vi "R1Master.vi"(6 "LabVIEW Web Service":refnum<class "Web Service.lvclass">=refnum) -> ()   [LabVIEW 2016]
uses:
  <vilib>/wsapi/Web Service.lvclass
  Controls/pH_SetParams Standard.ctl
  Controls/R1SBR_SetParams.ctl
  <vilib>/Platform/TimedLoop/XDataNode/timing_clust.ctl
  <vilib>/Platform/TimedLoop/XDataNode/nitl_modes.ctl
  <vilib>/Platform/TimedLoop/XDataNode/wakeup.ctl
  Controls/pH_Manual Standard.ctl
  <vilib>/Platform/TimedLoop/XDataNode/loadnilvce.vi
  <vilib>/Platform/TimedLoop/XDataNode/XDataNode.xnode
  <vilib>/Platform/TimedLoop/XDataNode/XDNodeRunTimeDep.lvlib
panel:
  out "ORP, V":dbl
  in  "R1SBR_SetParams":T1=[{"Phase"="Plug Feed", "Time, min"=60.0, "SBR_Manual"={"Media Pump"=TRUE, "Water Pump"=TRUE, "Effluent Pump"=FALSE, "Release Valve"=FALSE, "Gas Pump"=FALSE}}, {"Phase"="Mixed Feed", "Time, min"=80.0, "SBR_Manual"={"Media Pump"=TRUE, "Water Pump"=TRUE, "Effluent Pump"=FALSE, "Release Valve"=FALSE, "Gas Pump"=TRUE}}, {"Phase"="Mixed W/O Feed", "Time, min"=0.0, "SBR_Manual"={"Media Pump"=FALSE, "Water Pump"=FALSE, "Effluent Pump"=FALSE, "Release Valve"=FALSE, "Gas Pump"=TRUE}}, {"Phase"="Settle", "Time, min"=10.0, "SBR_Manual"={"Media Pump"=FALSE, "Water Pump"=FALSE, "Effluent Pump"=FALSE, "Release Valve"=FALSE, "Gas Pump"=FALSE}}, {"Phase"="Decant", "Time, min"=4.0, "SBR_Manual"={"Media Pump"=FALSE, "Water Pump"=FALSE, "Effluent Pump"=TRUE, "Release Valve"=TRUE, "Gas Pump"=FALSE}}, {"Phase"="Idle", "Time, min"=1.0, "SBR_Manual"={"Media Pump"=FALSE, "Water Pump"=FALSE, "Effluent Pump"=FALSE, "Release Valve"=FALSE, "Gas Pump"=FALSE}}] {"Time, min" min=1.0}
  out "error out Na":errorcluster
  out "error Out NH4 Nh4":errorcluster
  out "error out":errorcluster
  out "replace with nh4 set params":T2={"Set Point, mg/L"=0.0, "Tolerance, mg/L"=0.05, "N2 Valve Gain"=5000.0, "Air Valve Gain"=1000.0}
  in  "R1NH4Manual":cluster{"NH4 Pump Flowrate, ml/min":dbl}
  out "replace with nh4 switch":bool=TRUE
  in  "R1DOSetParams 2":T2={"Set Point, mg/L"=0.0, "Tolerance, mg/L"=0.05, "N2 Valve Gain"=5000.0, "Air Valve Gain"=1000.0}
  in  "R1 NH4_Switch":bool=TRUE
  out "add NH4 NA probes":cluster{"Signal":dbl, "Value":dbl}={"Signal"=0.0006045842747169349, "Value"=-0.0019895042131602755}
  out "error out (DATA COLLECT)":errorcluster
  out "error out (SBR)":errorcluster
  out "Graph":T3(graph)={"Value"=-0.0019895042131602755, "Value, UNITS HERE"=0.0, "Value"=8.00229484709635}
  in  "R1SBRManual":T4
  in  "R1 SBR_Switch":bool
  in  "R1DOSetParams":T2={"Set Point, mg/L"=0.25, "Tolerance, mg/L"=0.025, "N2 Valve Gain"=200.0, "Air Valve Gain"=1050.0}
  in  "R1DOManual":cluster{"Air MFC":dbl, "N2 MFC":dbl} {"Air MFC" scale=0.0..500.0; "N2 MFC" scale=0.0..500.0}
  in  "R1 DO_Switch":bool=TRUE
  out "R1DO":cluster{"Signal":dbl, "Value":dbl}={"Signal"=0.0006045842747169349, "Value"=-0.0019895042131602755}
  in  "R1 pH_Switch":bool=TRUE
  in  "R1pH_SetParams":T5={"Set Point"=8.0, "Tolerance"=0.1, "Pump Time On, secs"=6.0}
  in  "R1pH_Manual":cluster{"Acid Pump":bool, "Base Pump":bool}
  out "pH":cluster{"Signal":dbl, "Value":dbl}={"Signal"=0.013505965504601244, "Value"=8.00229484709635}
  out "Timestamp":string="03/16/2018 18:24:55.540"
  out "Status":string="Off"
  out "Cycle Time Elapsed":dbl
  out "Phase Time Elapsed":dbl
  # "Don't press the run button!"
  # "Use the web service input terminal to call the VIs on the Service subpalette of the Web Services palette. Do not remove it from the connector pane unless you don't need access to the palette."
  # "Any additional terminals added to the connector pane of a startup VI will be ignored."
  # "Don't press the run button!"
  # "SBR Control"
  # "If On, Automate SBR Cycle"
  # "DO Control"
  # "pH Control"
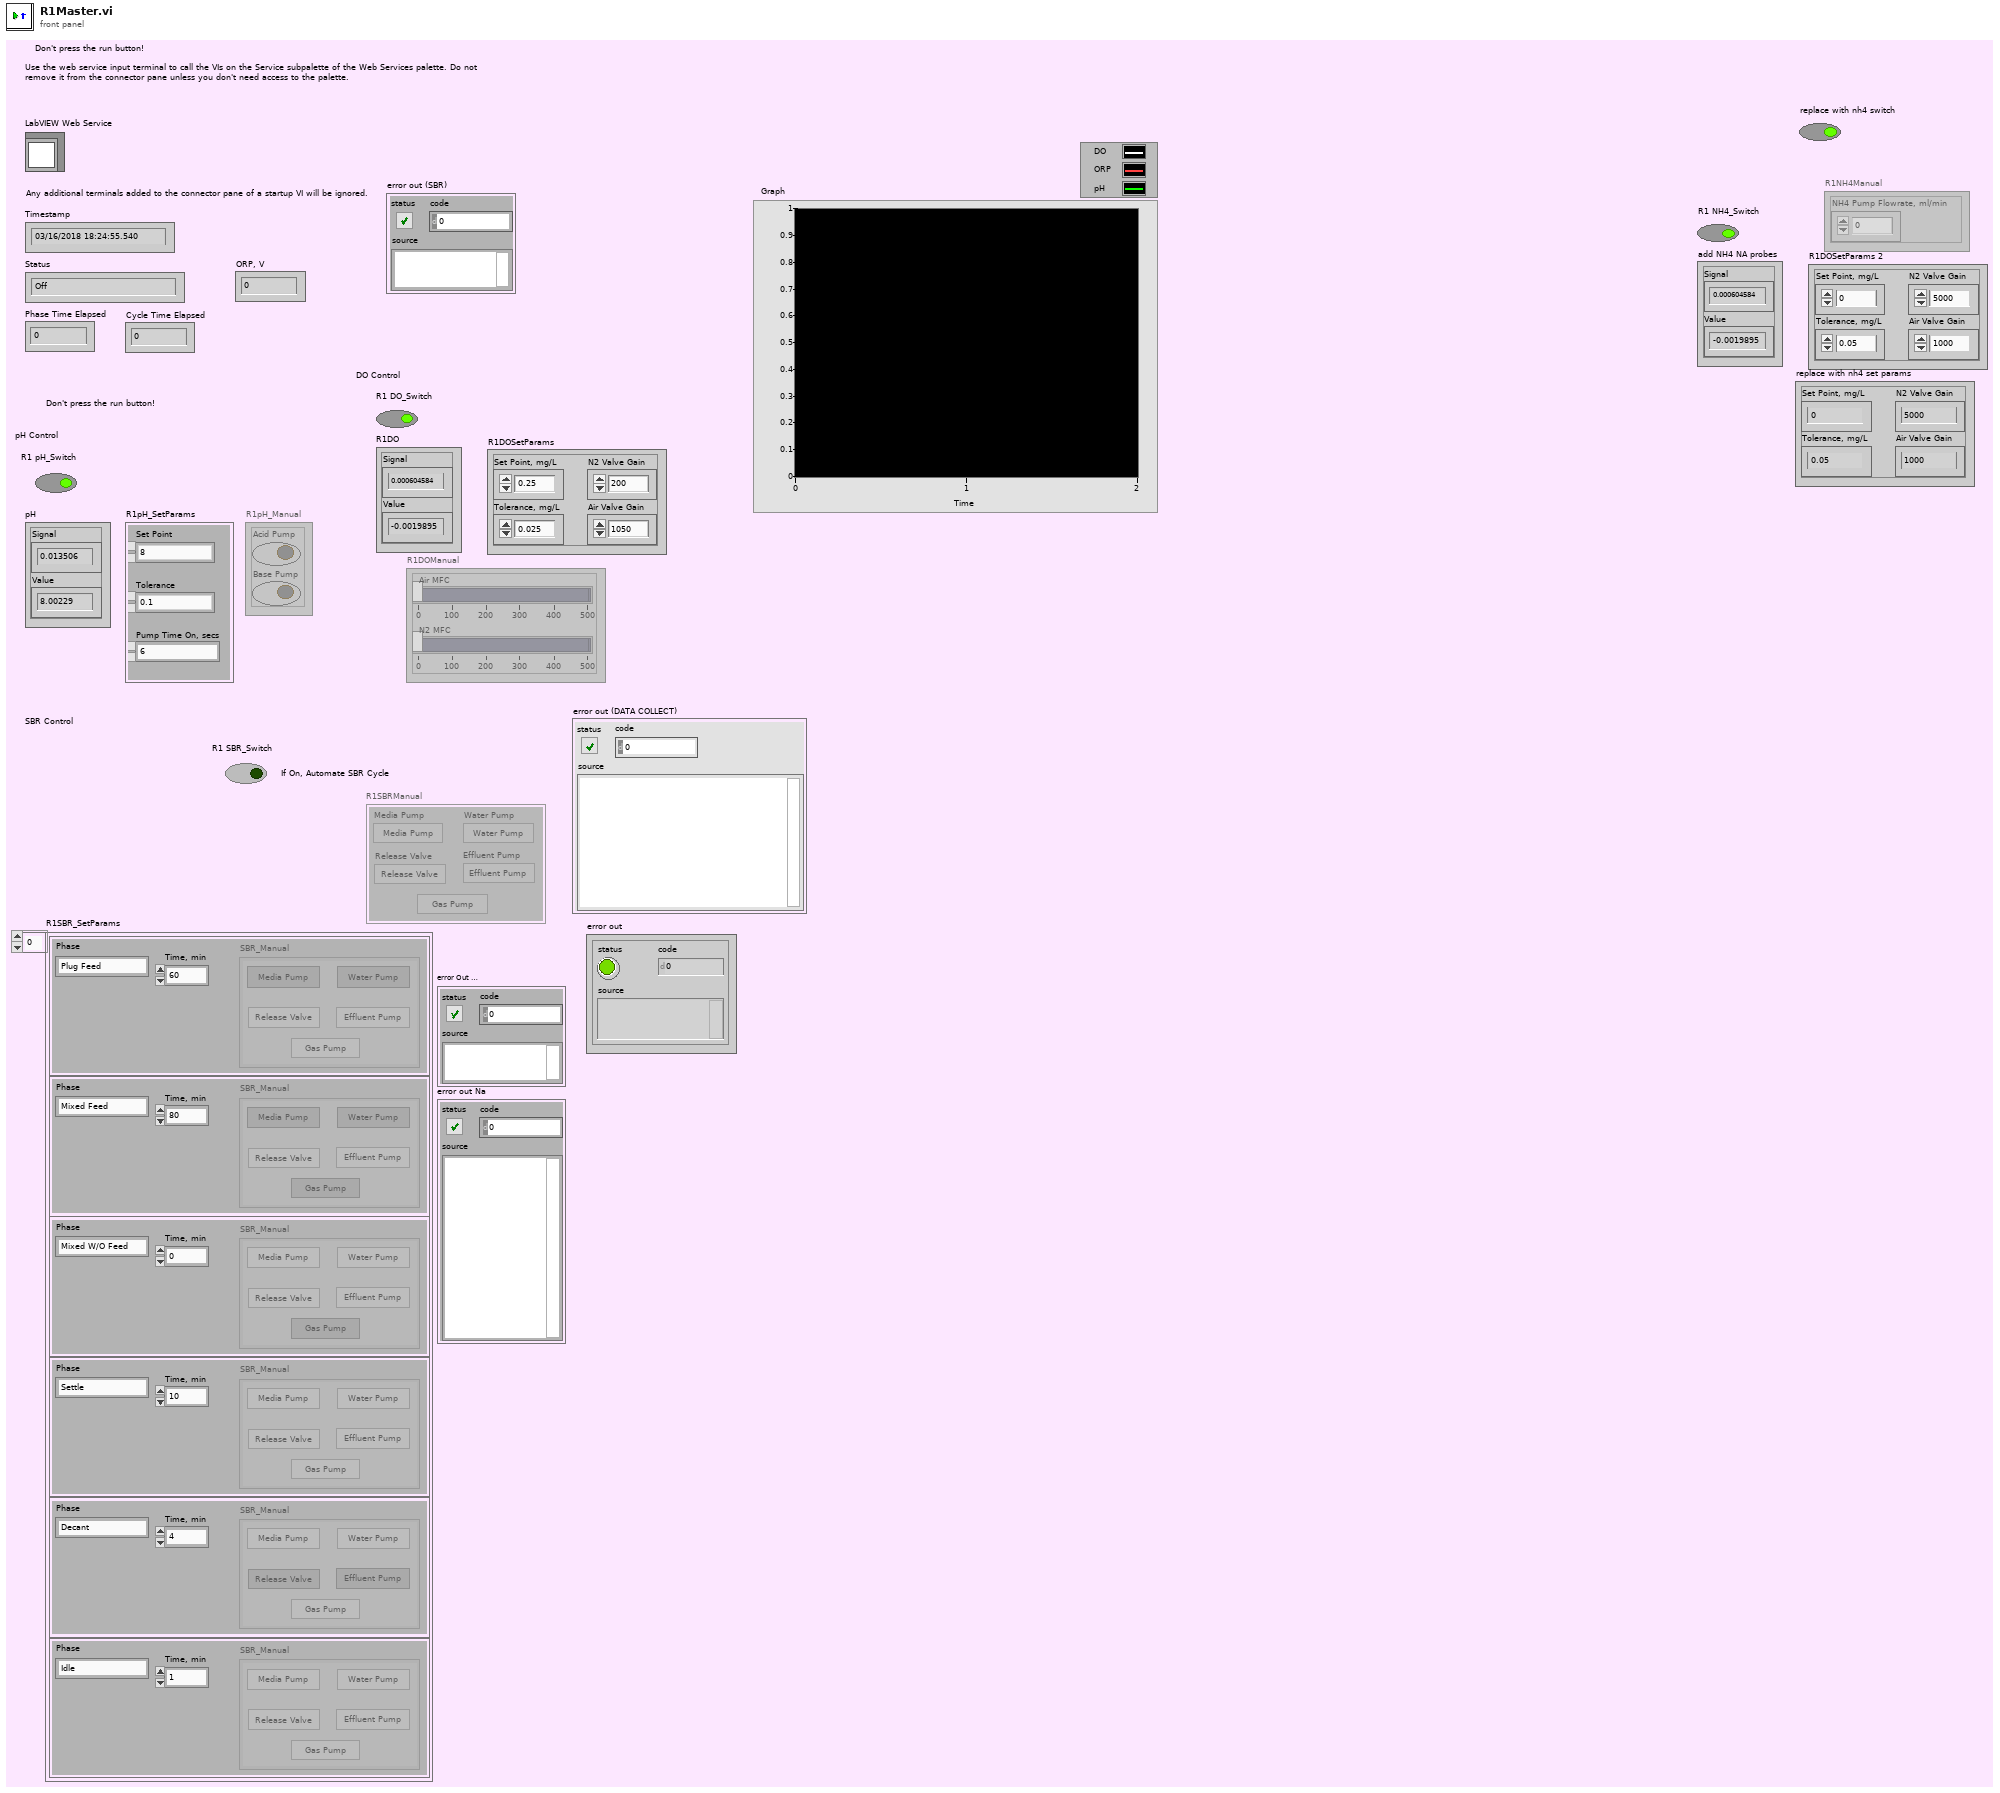
[diagram p1: front panel]
types:
  T1 = typedef "R1SBR_SetParams.ctl" = cluster{"Phase":string, "Time, min":dbl, "SBR_Manual":cluster{"Media Pump":bool, "Water Pump":bool, "Effluent Pump":bool, "Release Valve":bool, "Gas Pump":bool}}[]
  T2 = cluster{"Set Point, mg/L":dbl, "Tolerance, mg/L":dbl, "N2 Valve Gain":dbl, "Air Valve Gain":dbl}
  T3 = cluster{"Value":dbl, "Value, UNITS HERE":dbl, "Value":dbl}
  T4 = cluster{"Media Pump":bool, "Water Pump":bool, "Effluent Pump":bool, "Release Valve":bool, "Gas Pump":bool}
  T5 = typedef "pH_SetParams Standard.ctl" = cluster{"Set Point":dbl, "Tolerance":dbl, "Pump Time On, secs":dbl}
  T6 = typedef "XDNodeRunTimeDep.lvlib/timing_clust.ctl" = cluster{"Expected End [f-1]":u64, "Actual End [f-1]":u64, "Finished Late? [f-1]":bool, "Expected End [i-1]":u64, "Actual End [i-1]":u64, "Finished Late? [i-1]":bool, "Expected Start [i]":u64, "Actual Start [i]":u64, "Expected Start [f]":u64, "Actual Start [f]":u64, "Source Name":string, "Structure Name":string, "Period":i64, "Deadline":i64, "Offset":i64, "Start":i64, "Priority":i32, "Timeout":i32, "Mode":T7, "Wakeup Reason":T8, "Error":errorcluster, "Source Type":string, "Secondary Source Type":string, "Global End Time":u64, "Global Start Time":u64, "Frame Duration":u64, "Iteration Duration":u64, "Assigned CPU":i32, "I/O Scan Engine Mode":u32}
  T7 = typedef "XDNodeRunTimeDep.lvlib/nitl_modes.ctl" = enum32{"No Change", "Process missed periods, maintain original phase", "Discard missed periods, maintain original phase", "Process missed periods, ignore original phase", "Discard missed periods, ignore original phase"}
  T8 = typedef "XDNodeRunTimeDep.lvlib/wakeup.ctl" = enum32{"Normal", "Aborted", "Asynchronous wakeup", "Timing source error", "Timed loop error", "Timeout"}
  T9 = enum8{"Enabled", "Disabled", "Disabled and Grayed Out"}
  T10 = typedef "pH_Manual Standard.ctl" = cluster{"Acid Pump":bool, "Base Pump":bool}
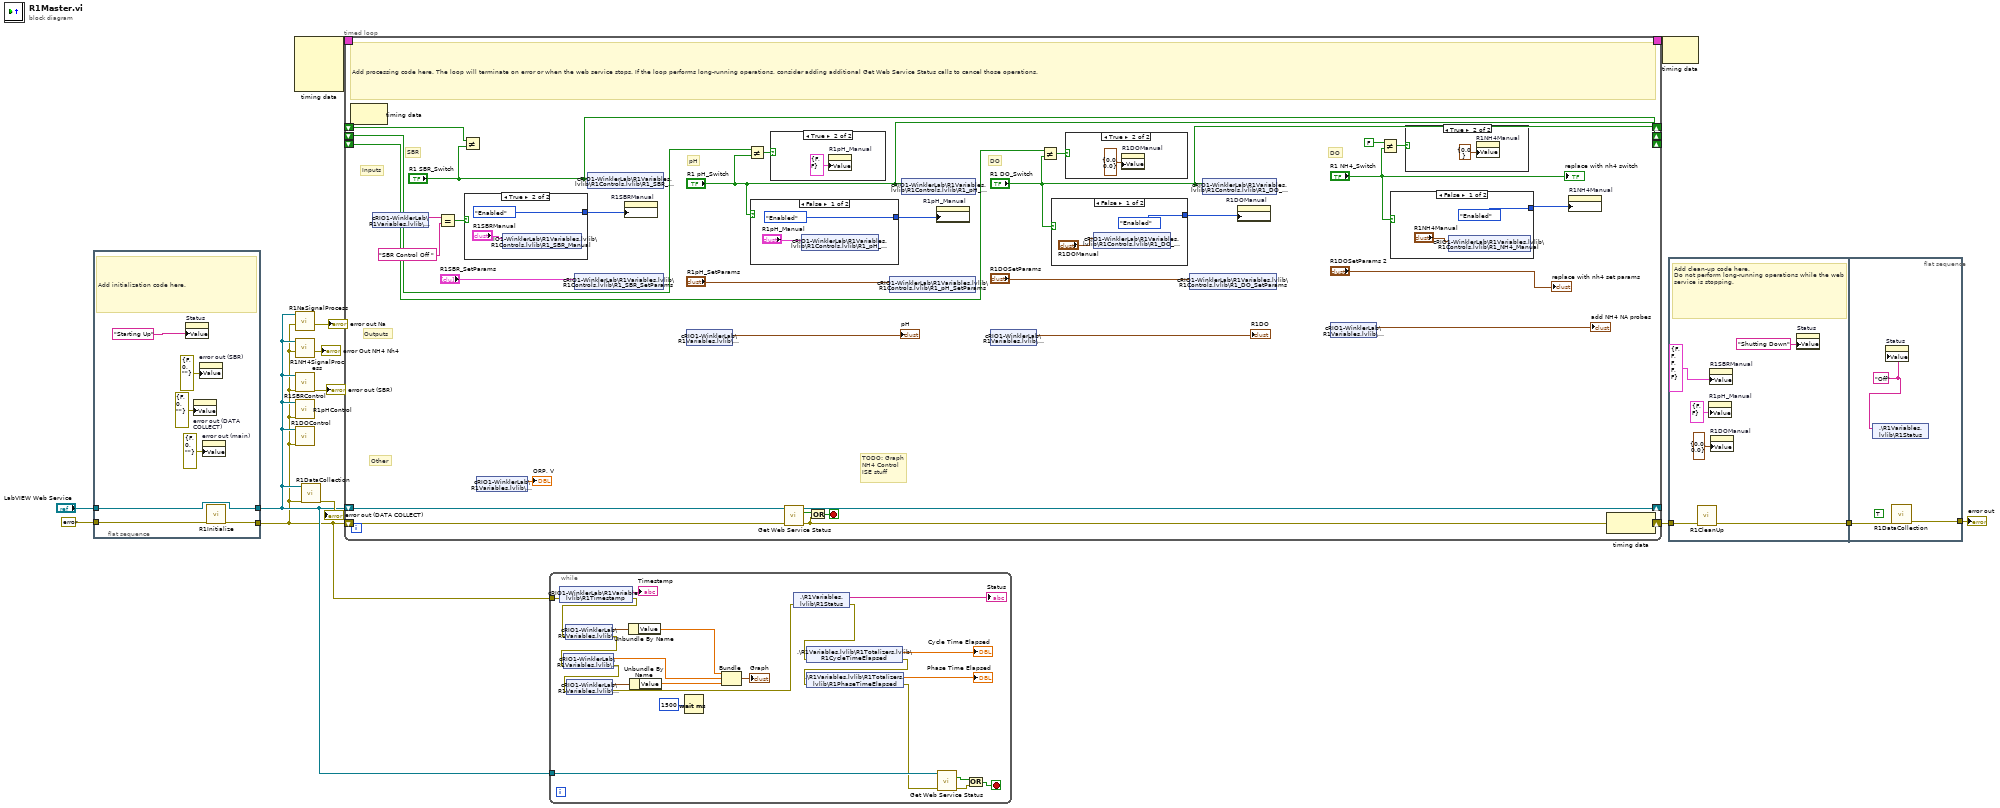
[diagram p0: block diagram]
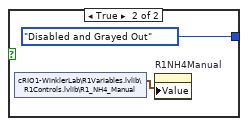
[diagram p3: hidden frame]
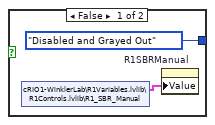
[diagram p6: hidden frame]
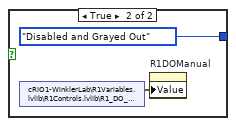
[diagram p7: hidden frame]
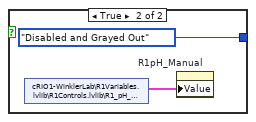
[diagram p8: hidden frame]
diagram:
  n1 = flat-sequence {
    tunnel: "LabVIEW Web Service" -> [w18]
    tunnel: errorcluster {"status"=FALSE, "code"=0, "source"=""} ("error constant") -> [w20]
    tunnel: [w19] -> w3
    tunnel: [w18] -> w4
    frame #0 {
      # "Add initialization code here."
      n2 = property on="Status" class="Str"("Value"="Starting Up" ("Status")) -> ()  [unwired: 2 in, 2 out]
      n3 = property on="error out (DATA COLLECT)" class="Clust (strict)"("Value"=errorcluster {"status"=FALSE, "code"=0, "source"=""} ("error out (DATA COLLECT)")) -> ()  [unwired: 2 in, 2 out]
      n4 = property on="error out (SBR)" class="Clust (strict)"("Value"=errorcluster {"status"=FALSE, "code"=0, "source"=""} ("error out (SBR)")) -> ()  [unwired: 2 in, 2 out]
      n5 = property on="error out (main)" class="Clust (strict)"("Value"=errorcluster {"status"=FALSE, "code"=0, "source"=""} ("error out")) -> ()  [unwired: 2 in, 2 out]
      n6 = call "R1Initialize.vi"("error in (no error)"=w20) -> ("error out"=w19:errorcluster)  [unwired: 10 in]
    }
  }
  n7 = node-c288() -> (w10:T6)  [unwired: 4 in]
  n8 = call "R1NaSignalProcess.vi"("error"=w3, "LabVIEW Web Service"=w4) -> ("error out"=→"error out Na":errorcluster)  [unwired: 9 in]
  n9 = call "R1NH4SignalProcess.vi"("error"=w3, "LabVIEW Web Service"=w4) -> ("error Out"=→"error Out NH4 Nh4":errorcluster)  [unwired: 9 in]
  n10 = call "R1SBRControl.vi"("error constant"=w3, "LabVIEW Web Service"=w4) -> ("error out"=→"error out (SBR)":errorcluster)  [unwired: 9 in]
  n11 = call "R1pHControl.vi"("error constant"=w3, "LabVIEW Web Service"=w4) -> ()  [unwired: 10 in]
  n12 = call "R1DOControl.vi"("error constant"=w3, "LabVIEW Web Service"=w4) -> ()  [unwired: 10 in]
  n13 = call "R1DataCollection.vi"("error constant"=w3, "LabVIEW Web Service"=w4) -> ("error out"=→"error out (DATA COLLECT)":errorcluster)  [unwired: 9 in]
  n14 = timed-loop {
    shift-right: [w50] -> w11
    shift-left: w3 -> [w49]
    shift-right: [w47] -> _
    shift-left: w4 -> [w47]
    timing: w10 -> [_]
    timing-out: [_] -> w9
    shift-right: ["R1 SBR_Switch"] -> _
    shift-left: _ -> [w23]
    shift-right: ["R1 pH_Switch"] -> _
    shift-left: _ -> [w38]
    shift-right: ["R1 DO_Switch"] -> _
    shift-left: _ -> [w36]
    stop <- w48 stop-if-true
    # "DO"
    # "TODO: Graph\nNH4 Control\nISE stuff"
    # "DO"
    # "pH"
    # "Other"
    # "Outputs"
    # "Inputs"
    # "SBR"
    # "Add processing code here. The loop will terminate on error or when the web service stops. If the loop performs long-running operations, consider adding additional Get Web Service Status calls to cancel those operations."
    n15 = node-c288() -> ()  [unwired: 1 in, 1 out]
    n16 = shared-variable "cRIO1-WinklerLab\\R1Variables.lvlib\\R1Status"() -> (w26:string)  [unwired: 1 in, 1 out]
    n17 = Equal?(x=w26, y="SBR Control Off " ("string")) -> (x = y?=w24:bool)
    n18 = Not Equal?(x=w23, y="R1 SBR_Switch") -> ()  [unwired: 1 out]
    n19 = case shown="True" w24 {
      tunnel: [T9."Disabled and Grayed Out" ("Disabled") T9."Enabled" ("Disabled")] -> w40
      frame False {
        n20 = shared-variable "cRIO1-WinklerLab\\R1Variables.lvlib\\R1Controls.lvlib\\R1_SBR_Manual"() -> (w59:T4)  [unwired: 1 in, 1 out]
        n21 = property on="R1SBRManual" class="Clust (strict)"("Value"=w59) -> ()  [unwired: 2 in, 2 out]
      }
      frame True {
        n22 = shared-variable "cRIO1-WinklerLab\\R1Variables.lvlib\\R1Controls.lvlib\\R1_SBR_Manual"("R1SBRManual") -> ()  [unwired: 1 in, 1 out]
      }
    }
    n23 = shared-variable "cRIO1-WinklerLab\\R1Variables.lvlib\\R1Signals.lvlib\\R1ORP"() -> (→"ORP, V":dbl)  [unwired: 1 in, 1 out]
    n24 = shared-variable "cRIO1-WinklerLab\\R1Variables.lvlib\\R1Controls.lvlib\\R1_SBR_SetParams"("R1SBR_SetParams") -> ()  [unwired: 1 in, 1 out]
    n25 = shared-variable "cRIO1-WinklerLab\\R1Variables.lvlib\\R1Controls.lvlib\\R1_SBR_Switch"("R1 SBR_Switch") -> ()  [unwired: 1 in, 1 out]
    n26 = property on="R1SBRManual" class="Clust (strict)"("DisabledEnum"=w40) -> ()  [unwired: 2 in, 2 out]
    n27 = shared-variable "cRIO1-WinklerLab\\R1Variables.lvlib\\R1Signals.lvlib\\R1pH"() -> (→"pH":cluster{"Signal":dbl, "Value":dbl})  [unwired: 1 in, 1 out]
    n28 = Not Equal?(x=w38, y="R1 pH_Switch") -> (x != y?=w37:bool)
    n29 = case shown="False" "R1 pH_Switch" {
      tunnel: [T9."Enabled" ("Disabled") T9."Disabled and Grayed Out" ("Disabled")] -> w45
      frame False {
        n30 = shared-variable "cRIO1-WinklerLab\\R1Variables.lvlib\\R1Controls.lvlib\\R1_pH_Manual"("R1pH_Manual") -> ()  [unwired: 1 in, 1 out]
      }
      frame True {
        n31 = shared-variable "cRIO1-WinklerLab\\R1Variables.lvlib\\R1Controls.lvlib\\R1_pH_Manual"() -> (w69:T10)  [unwired: 1 in, 1 out]
        n32 = property on="R1pH_Manual" class="Clust (strict)"("Value"=w69) -> ()  [unwired: 2 in, 2 out]
      }
    }
    n33 = case shown="True" w37 {
      frame False {
      }
      frame True {
        n34 = property on="R1pH_Manual" class="Clust (strict)"("Value"=cluster{"Acid Pump":bool, "Base Pump":bool} {"Acid Pump"=FALSE, "Base Pump"=FALSE} ("R1pH_Manual")) -> ()  [unwired: 2 in, 2 out]
      }
    }
    n35 = call <vilib>:"Get Web Service Status.vi"("LabVIEW Web Service"=w47, "error in (no error)"=w49) -> ("service stopping?"=w51:bool, "error out"=w50:errorcluster)  [unwired: 11 in, 1 out]
    n36 = Or(x=w51, y=w50) -> (x .or. y?=w48:bool)
    n37 = shared-variable "cRIO1-WinklerLab\\R1Variables.lvlib\\R1Controls.lvlib\\R1_pH_SetParams"("R1pH_SetParams") -> ()  [unwired: 1 in, 1 out]
    n38 = shared-variable "cRIO1-WinklerLab\\R1Variables.lvlib\\R1Controls.lvlib\\R1_pH_Switch"("R1 pH_Switch") -> ()  [unwired: 1 in, 1 out]
    n39 = property on="R1pH_Manual" class="Clust (strict)"("DisabledEnum"=w45) -> ()  [unwired: 2 in, 2 out]
    n40 = shared-variable "cRIO1-WinklerLab\\R1Variables.lvlib\\R1Signals.lvlib\\R1DO"() -> (→"R1DO":cluster{"Signal":dbl, "Value":dbl})  [unwired: 1 in, 1 out]
    n41 = Not Equal?(x=w36, y="R1 DO_Switch") -> (x != y?=w35:bool)
    n42 = case shown="False" "R1 DO_Switch" {
      tunnel: [T9."Enabled" ("Disabled") T9."Disabled and Grayed Out" ("Disabled")] -> w42
      frame False {
        n43 = shared-variable "cRIO1-WinklerLab\\R1Variables.lvlib\\R1Controls.lvlib\\R1_DO_Manual"("R1DOManual") -> ()  [unwired: 1 in, 1 out]
      }
      frame True {
        n44 = shared-variable "cRIO1-WinklerLab\\R1Variables.lvlib\\R1Controls.lvlib\\R1_DO_Manual"() -> (w65:cluster{"Air MFC":dbl, "N2 MFC":dbl})  [unwired: 1 in, 1 out]
        n45 = property on="R1DOManual" class="Clust (strict)"("Value"=w65) -> ()  [unwired: 2 in, 2 out]
      }
    }
    n46 = case shown="True" w35 {
      frame False {
      }
      frame True {
        n47 = property on="R1DOManual" class="Clust (strict)"("Value"=cluster{"Air MFC":dbl, "N2 MFC":dbl} {"Air MFC"=0.0, "N2 MFC"=0.0} ("R1DOManual")) -> ()  [unwired: 2 in, 2 out]
      }
    }
    n48 = shared-variable "cRIO1-WinklerLab\\R1Variables.lvlib\\R1Controls.lvlib\\R1_DO_SetParams"("R1DOSetParams") -> ()  [unwired: 1 in, 1 out]
    n49 = shared-variable "cRIO1-WinklerLab\\R1Variables.lvlib\\R1Controls.lvlib\\R1_DO_Switch"("R1 DO_Switch") -> ()  [unwired: 1 in, 1 out]
    n50 = property on="R1DOManual" class="Clust (strict)"("DisabledEnum"=w42) -> ()  [unwired: 2 in, 2 out]
    n51 = shared-variable "cRIO1-WinklerLab\\R1Variables.lvlib\\R1Signals.lvlib\\R1DO"() -> (→"add NH4 NA probes":cluster{"Signal":dbl, "Value":dbl})  [unwired: 1 in, 1 out]
    n52 = Not Equal?(x=FALSE, y="R1 NH4_Switch") -> (x != y?=w32:bool)
    n53 = case shown="False" "R1 NH4_Switch" {
      tunnel: [T9."Enabled" ("Disabled") T9."Disabled and Grayed Out" ("Disabled")] -> w28
      frame False {
        n54 = shared-variable "cRIO1-WinklerLab\\R1Variables.lvlib\\R1Controls.lvlib\\R1_NH4_Manual"("R1NH4Manual") -> ()  [unwired: 1 in, 1 out]
      }
      frame True {
        n55 = shared-variable "cRIO1-WinklerLab\\R1Variables.lvlib\\R1Controls.lvlib\\R1_NH4_Manual"() -> (w55:cluster{"NH4 Pump Flowrate, ml/min":dbl})  [unwired: 1 in, 1 out]
        n56 = property on="R1NH4Manual" class="Clust (strict)"("Value"=w55) -> ()  [unwired: 2 in, 2 out]
      }
    }
    n57 = case shown="True" w32 {
      frame False {
      }
      frame True {
        n58 = property on="R1NH4Manual" class="Clust (strict)"("Value"=cluster{"NH4 Pump Flowrate, ml/min":dbl} {"NH4 Pump Flowrate, ml/min"=0.0} ("R1NH4Manual")) -> ()  [unwired: 2 in, 2 out]
      }
    }
    n59 = property on="R1NH4Manual" class="Clust (strict)"("DisabledEnum"=w28) -> ()  [unwired: 2 in, 2 out]
    n60 = node-c288() -> ()  [unwired: 1 in, 1 out]
    "replace with nh4 switch" <- "R1 NH4_Switch"
    "replace with nh4 set params" <- "R1DOSetParams 2"
  }
  n61 = while {
    tunnel: w4 -> [w90]
    tunnel: w3 -> [w81]
    stop <- w87 stop-if-true
    n62 = shared-variable "cRIO1-WinklerLab\\R1Variables.lvlib\\R1Timestamp"(error in=w81) -> (→"Timestamp":string, error out=w80:errorcluster)
    n63 = shared-variable "cRIO1-WinklerLab\\R1Variables.lvlib\\R1Signals.lvlib\\R1DO"(error in=w80) -> (w91:cluster{"Signal":dbl, "Value":dbl}, error out=w79:errorcluster)
    n64 = shared-variable "cRIO1-WinklerLab\\R1Variables.lvlib\\R1Signals.lvlib\\R1ORP"(error in=w79) -> (w73:dbl, error out=w78:errorcluster)
    n65 = shared-variable "cRIO1-WinklerLab\\R1Variables.lvlib\\R1Signals.lvlib\\R1pH"(error in=w78) -> (w92:cluster{"Signal":dbl, "Value":dbl}, error out=w77:errorcluster)
    n66 = Unbundle By Name(w91) -> ("Value"=w93:dbl)
    n67 = Unbundle By Name(w92) -> ("Value"=w94:dbl)
    n68 = Wait (ms)(milliseconds to wait=u32 1500) -> ()  [unwired: 1 out]
    n69 = Bundle("Value"=w93, "Double"=w73, "Value"=w94) -> (→"Graph":cluster{"Value":dbl, "Double":dbl, "Value":dbl})  [unwired: 1 in]
    n70 = shared-variable ".\\R1Variables.lvlib\\R1Status"(error in=w77) -> (→"Status":string, error out=w76:errorcluster)
    n71 = shared-variable ".\\R1Variables.lvlib\\R1Totalizers.lvlib\\R1CycleTimeElapsed"(error in=w76) -> (→"Cycle Time Elapsed":dbl, error out=w75:errorcluster)
    n72 = shared-variable ".\\R1Variables.lvlib\\R1Totalizers.lvlib\\R1PhaseTimeElapsed"(error in=w75) -> (→"Phase Time Elapsed":dbl, error out=w74:errorcluster)
    n73 = call <vilib>:"Get Web Service Status.vi"("LabVIEW Web Service"=w90, "error in (no error)"=w74) -> ("service stopping?"=w89:bool, "error out"=w88:errorcluster)  [unwired: 11 in, 1 out]
    n74 = Or(x=w89, y=w88) -> (x .or. y?=w87:bool)
  }
  n75 = node-c288(w9) -> ()  [unwired: 1 out]
  n76 = flat-sequence {
    tunnel: w11 -> [w99]
    tunnel: [w98] -> w7
    tunnel: w7 -> [w104]
    tunnel: [w103] -> w6
    frame #0 {
      # "Add clean-up code here.\nDo not perform long-running operations while the web service is stopping."
      n77 = call "R1CleanUp.vi"("error in (no error)"=w99) -> ("error out"=w98:errorcluster)  [unwired: 10 in]
      n78 = property on="R1pH_Manual" class="Clust (strict)"("Value"=cluster{"Acid Pump":bool, "Base Pump":bool} {"Acid Pump"=FALSE, "Base Pump"=FALSE} ("R1pH_Manual")) -> ()  [unwired: 2 in, 2 out]
      n79 = property on="R1SBRManual" class="Clust (strict)"("Value"=T4 {"Media Pump"=FALSE, "Water Pump"=FALSE, "Effluent Pump"=FALSE, "Release Valve"=FALSE, "Gas Pump"=FALSE} ("R1SBRManual")) -> ()  [unwired: 2 in, 2 out]
      n80 = property on="R1DOManual" class="Clust (strict)"("Value"=cluster{"Air MFC":dbl, "N2 MFC":dbl} {"Air MFC"=0.0, "N2 MFC"=0.0} ("R1DOManual")) -> ()  [unwired: 2 in, 2 out]
      n81 = property on="Status" class="Str"("Value"="Shutting Down" ("Status")) -> ()  [unwired: 2 in, 2 out]
    }
    frame #1 {
      w102 = "Off" ("Status")
      (unwired) TRUE ("Write Once")
      n82 = shared-variable ".\\R1Variables.lvlib\\R1Status"(w102) -> ()  [unwired: 1 in, 1 out]
      n83 = property on="Status" class="Str"("Value"=w102) -> ()  [unwired: 2 in, 2 out]
      n84 = call "R1DataCollection.vi"("error constant"=w104) -> ("error out"=w103:errorcluster)  [unwired: 10 in]
    }
  }
  "error out" <- w6
